vi "CMD_SETVAC.vi"(6 "Gantry in":refnum<class "Gantry Class.lvclass">, 8 "error in (no error)":errorcluster, 10 "Arguments":string[](array[string]), 11 "gScript Interpreter in":refnum<class "gScript Interpreter.lvclass">) -> (0 "error out":errorcluster, 3 "gScript Interpreter out":refnum<class "gScript Interpreter.lvclass">, 4 "Gantry out":refnum<class "Gantry Class.lvclass">)   [LabVIEW 2017, in "gScript Interpreter.lvclass"]
uses:
  gScript Interpreter.lvclass
  Shared Components/Gantry Class/Gantry Class.lvclass
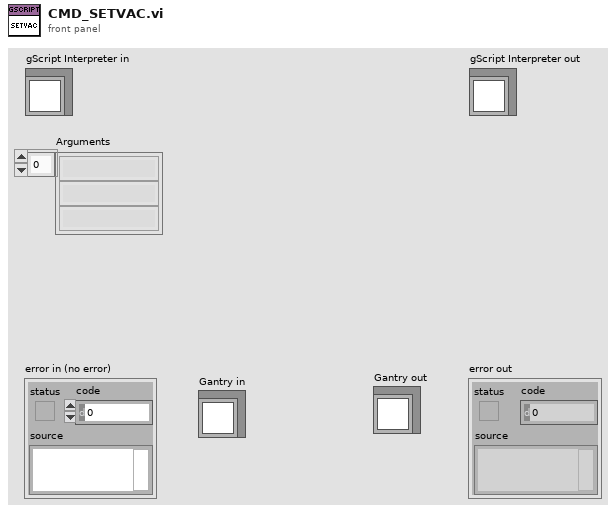
[diagram p1: front panel]
types:
  T1 = typedef "Memory Cell.ctl" = cluster{"type":T2, "x":dbl, "y":dbl, "z":dbl, "w":dbl}
  T2 = typedef "Memory Cell Type Enum.ctl" = enum16{"integer", "float", "vector", "rotation"}
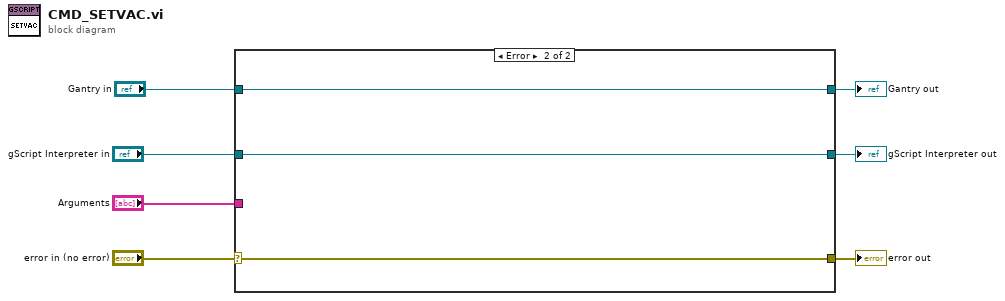
[diagram p0: block diagram]
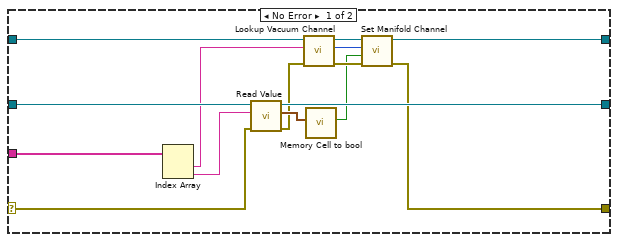
[diagram p2: hidden frame]
diagram:
  n1 = case shown="Error" "error in (no error)" {
    selector: "error in (no error)" -> [w19 w25]
    tunnel: [w8 w25] -> w6
    tunnel: [w16 w24] -> w4
    tunnel: "gScript Interpreter in" -> [w21 w24]
    tunnel: "Arguments" -> [w22 _]
    tunnel: "Gantry in" -> [w18 w23]
    tunnel: [w9 w23] -> w1
    frame No Error {
      n2 = Index Array(array=w22) -> (element #1=w14:string, element #2=w20:string)  [unwired: 2 in]
      n3 = call-dynamic "Read Value.vi"("error in (no error)"=w19, "String in"=w20, "gScript Interpreter in"=w21) -> ("error out"=w15:errorcluster, "Memory Cell"=w17:T1, "gScript Interpreter out"=w16:refnum<class "gScript Interpreter.lvclass">)  [unwired: 6 in]
      n4 = call-dynamic "Lookup Vacuum Channel.vi"("error in (no error)"=w15, "String"=w14, "Gantry Class in"=w18) -> ("error out"=w12:errorcluster, "Channel Number"=w11:i32, "Gantry Class out"=w13:refnum<class "Gantry Class.lvclass">)  [unwired: 5 in]
      n5 = call "Memory Cell to bool.vi"("Memory Cell"=w17) -> ("bool out"=w10:bool)  [unwired: 10 in]
      n6 = call-dynamic "Set Manifold Channel.vi"("error in"=w12, "On/Off"=w10, "Manifold Channel"=w11, "Gantry in"=w13) -> ("error out"=w8:errorcluster, "Gantry out"=w9:refnum<class "Gantry Class.lvclass">)  [unwired: 6 in]
    }
    frame Error {
    }
  }
  "error out" <- w6
  "gScript Interpreter out" <- w4
  "Gantry out" <- w1
